vi "single-axis scan data.vi"(8 "Error In":errorcluster, 9 "Data to append":cluster{"Position":dbl, "averaged values":dbl[]}, 10 "scan data Input":T1, 11 "action (R)":T2=enum."read") -> (0 "Error out":errorcluster, 2 "scan data output":T1)   [LabVIEW 2011]
doc: "Functional Global Variable for the algorithm settings. The used method as well as the max. Iteration steps and the tolerance can be given. In addition, the algorithm can be told to use boundaries (if possible)."
uses:
  controls/scan data action.ctl
  controls/single-axis scan data.ctl
panel:
  # "Input"
  # "Output"
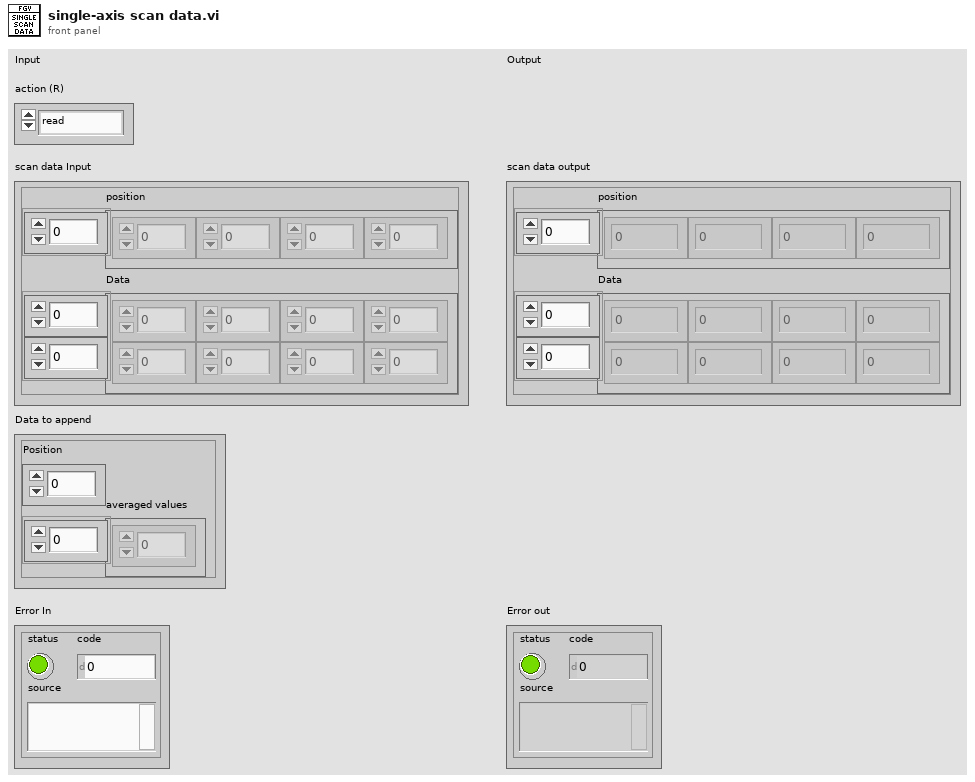
[diagram p1: front panel]
types:
  T1 = typedef "single-axis scan data.ctl" = cluster{"position":dbl[], "Data":dbl[][]}
  T2 = typedef "scan data action.ctl" = enum16{"initialize", "append", "read", "write"}
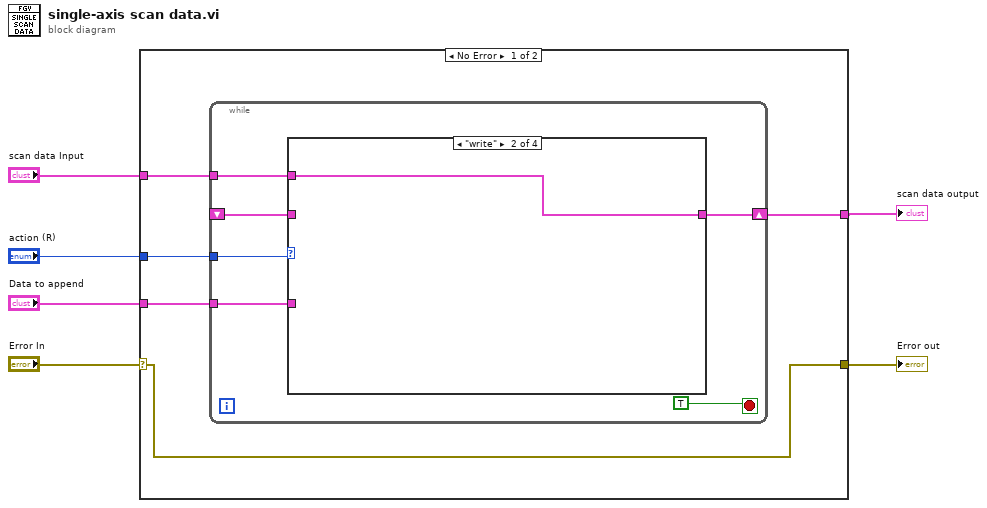
[diagram p0: block diagram]
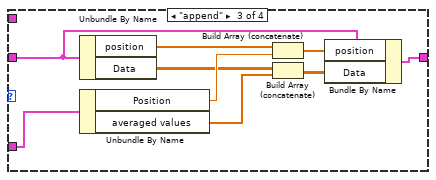
[diagram p3: hidden frame]
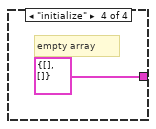
[diagram p4: hidden frame]
diagram:
  n1 = case shown="No Error" "Error In" {
    selector: "Error In" -> [w8 w31]
    tunnel: "action (R)" -> [w11 _]
    tunnel: [w8 w31] -> w4
    tunnel: "scan data Input" -> [w10 w30]
    tunnel: [w9 w30] -> w1
    tunnel: "Data to append" -> [w7 _]
    frame No Error {
      n2 = while {
        tunnel: w11 -> [w16]
        tunnel: w10 -> [w15]
        shift-right: [w13] -> w9
        shift-left: _ -> [w14]
        tunnel: w7 -> [w12]
        stop <- TRUE stop-if-true
        n3 = case shown="\"write\"" w16 {
          tunnel: w15 -> [_ w19 _ _]
          tunnel: w14 -> [w18 _ w20 _]
          tunnel: [w18 w19 w21 T1 {"position"=[], "Data"=[]} ("scan data Input")] -> w13
          tunnel: w12 -> [_ _ w28 _]
          frame "read", Default {
          }
          frame "write" {
          }
          frame "append" {
            n4 = Unbundle By Name(w20) -> ("position"=w26:dbl[], "Data"=w25:dbl[][])
            n5 = Unbundle By Name(w28) -> ("Position"=w27:dbl, "averaged values"=w24:dbl[])
            n6 = Build Array (concatenate)(w26, w27) -> (w22:dbl[])
            n7 = Build Array (concatenate)(w25, w24) -> (w23:dbl[][])
            n8 = Bundle By Name(cluster=w20, "position"=w22, "Data"=w23) -> (w21:T1)
          }
          frame "initialize" {
            # "empty array"
          }
        }
      }
    }
    frame Error {
    }
  }
  "Error out" <- w4
  "scan data output" <- w1
